vi "Implement Dynamic Dispatch VIs.vi"(8 "error in (no error)":errorcluster, 11 "Mock Class Generator In":refnum<class "Mock Class Generator.lvclass">) -> (0 "error out":errorcluster, 3 "Mock Class Generator Out":refnum<class "Mock Class Generator.lvclass">)   [LabVIEW 2020, in "Mock Class Generator.lvclass"]
uses:
  Mock Class Generator.lvclass
  Mock Class Generator.lvclass/Mock Class Generator.ctl
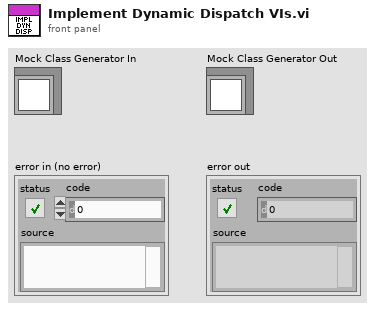
[diagram p1: front panel]
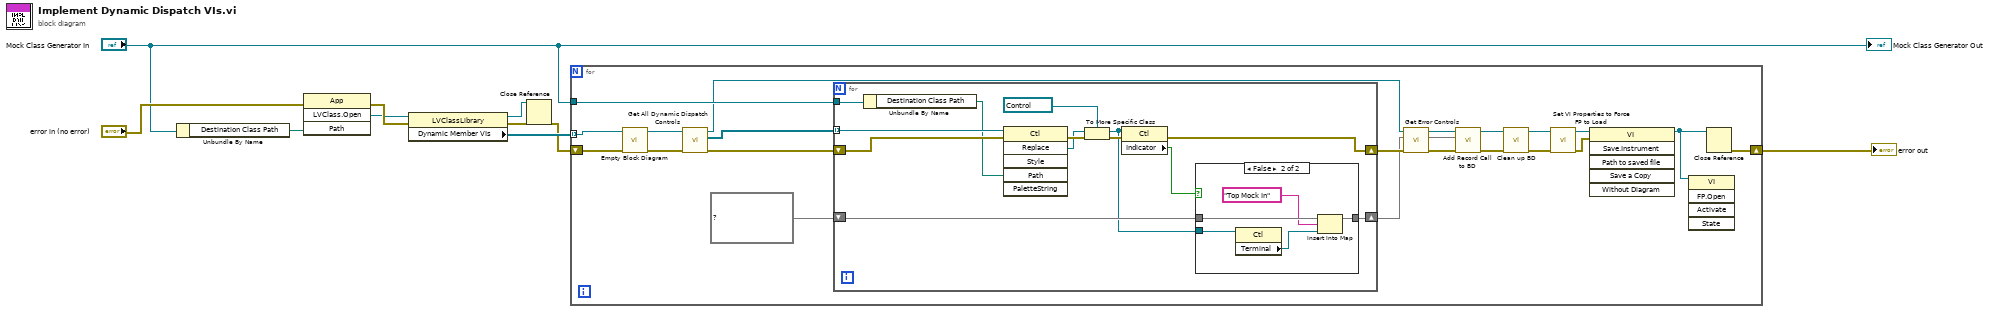
[diagram p0: block diagram]
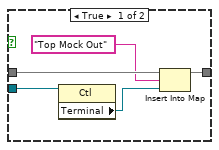
[diagram p2: hidden frame]
diagram:
  n1 = Unbundle By Name("Mock Class Generator In") -> ("Destination Class Path"=w10:path)
  n2 = invoke class="App" method="LVClass.Open"(error in="error in (no error)", "Path"=w10) -> (error out=w9:errorcluster, "LVClass.Open"=w4:refnum<vi>)  [unwired: 2 in, 2 out]
  n3 = property class="LVClassLibrary"(reference=w4, error in=w9) -> (reference out=w5:refnum<vi>, error out=w6:errorcluster, "Dynamic Member VIs"=w7:refnum<vi>[])
  n4 = Close Reference(reference=w5, error in (no error)=w6) -> (error out=w3:errorcluster)
  n5 = for {
    tunnel: w7 -> [w16] mode=indexing
    tunnel: "Mock Class Generator In" -> [w31]
    shift-right: [w29] -> w1
    shift-left: w3 -> [w11]
    n6 = call "Empty Block Diagram.vi"("error in (no error)"=w11, "VI in"=w16) -> ("error out"=w12:errorcluster, "reference out"=w28:refnum<vi>)  [unwired: 8 in]
    n7 = call "Get All Dynamic Dispatch Controls.vi"("error in (no error)"=w12, "VI in"=w28) -> ("error out"=w32:errorcluster, "Dynamic Dispatch Controls"=w30:refnum<vi>[], "reference out"=w26:refnum<vi>)  [unwired: 7 in]
    n8 = for {
      tunnel: w30 -> [w45] mode=indexing
      shift-right: [w37] -> w27
      shift-left: w32 -> [w44]
      tunnel: w31 -> [w43]
      shift-right: [w35] -> w22
      shift-left: map{string, refnum<vi>} {} ("map") -> [w36]
      n9 = Unbundle By Name(w43) -> ("Destination Class Path"=w42:path)
      n10 = invoke class="Ctl" method="Replace"(reference=w45, error in=w44, "Path"=w42) -> (error out=w41:errorcluster, "Replace"=w39:refnum<vi>)  [unwired: 3 in, 4 out]
      n11 = To More Specific Class(target class=refnum<vi> refnum ("reference out"), reference=w39, error in=w41) -> (specific class reference=w33:refnum<vi>, error out=w40:errorcluster)
      n12 = property class="Ctl"(reference=w33, error in=w40) -> (error out=w37:errorcluster, "Indicator"=w34:bool)  [unwired: 1 out]
      n13 = case shown="False" w34 {
        tunnel: w36 -> [w50 w55]
        tunnel: [w49 w54] -> w35
        tunnel: w33 -> [w47 w52]
        frame True {
          n14 = property class="Ctl"(reference=w47) -> ("Terminal"=w46:refnum<vi>)  [unwired: 1 in, 2 out]
          n15 = Insert Into Map(map in=w50, key="Top Mock Out", value=w46) -> (map out=w49:map{string, refnum<vi>})  [unwired: 2 out]
        }
        frame False {
          n16 = property class="Ctl"(reference=w52) -> ("Terminal"=w51:refnum<vi>)  [unwired: 1 in, 2 out]
          n17 = Insert Into Map(map in=w55, key="Top Mock In", value=w51) -> (map out=w54:map{string, refnum<vi>})  [unwired: 2 out]
        }
      }
    }
    n18 = call "Get Error Controls.vi"("error in (no error)"=w27, "map"=w22, "VI in"=w26) -> ("error out"=w24:errorcluster, "map out"=w21:map{string, refnum<vi>}, "reference out"=w25:refnum<vi>)  [unwired: 6 in]
    n19 = call "Add Record Call to BD.vi"("error in (no error)"=w24, "map"=w21, "VI in"=w25) -> ("error out"=w13:errorcluster, "VI out"=w20:refnum<vi>)  [unwired: 7 in]
    n20 = call "Clean up BD.vi"("error in (no error)"=w13, "VI in"=w20) -> ("error out"=w14:errorcluster, "VI out"=w19:refnum<vi>)  [unwired: 8 in]
    n21 = call "Set VI Properties to Force FP to Load.vi"("error in (no error)"=w14, "VI in"=w19) -> ("error out"=w15:errorcluster, "VI out"=w17:refnum<vi>)  [unwired: 8 in]
    n22 = invoke class="VI" method="Save.Instrument"(reference=w17, error in=w15) -> (reference out=w18:refnum<vi>)  [unwired: 4 in, 5 out]
    n23 = invoke class="VI" method="FP.Open"(reference=w18) -> ()  [unwired: 4 in, 5 out]
    n24 = Close Reference(reference=w18) -> (error out=w29:errorcluster)  [unwired: 1 in]
  }
  "error out" <- w1
  "Mock Class Generator Out" <- "Mock Class Generator In"
